vi "Build Array SB.vi"() -> ()   [LabVIEW 2019]
panel:
  out "Output Array":dbl[](array[numeric])
  in  "Index":i32
  in  "Element to Insert":dbl
  in  "Insert":bool
  in  "Stop":bool
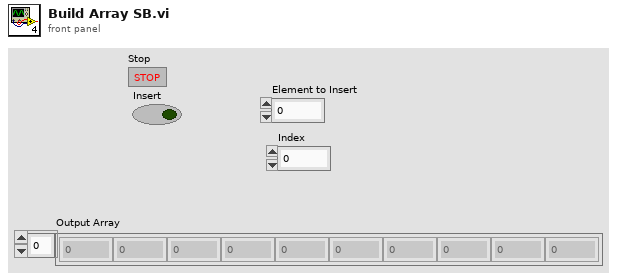
[diagram p1: front panel]
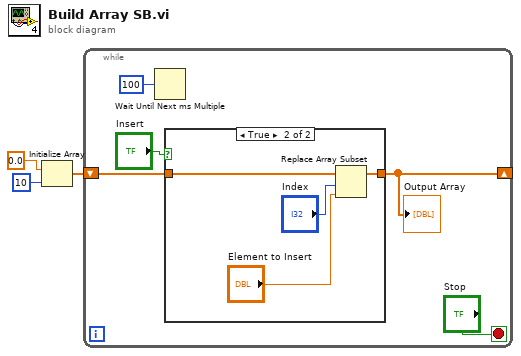
[diagram p0: block diagram]
diagram:
  n1 = Initialize Array(0.0 ("element"), 10 ("dimension size")) -> (w3:dbl[])
  n2 = while {
    shift-right: [w4] -> _
    shift-left: w3 -> [w5]
    stop <- "Stop" stop-if-true
    n3 = Wait Until Next ms Multiple(millisecond multiple=u32 100) -> ()  [unwired: 1 out]
    n4 = case shown="True" "Insert" {
      tunnel: [w9 w13] -> w4
      tunnel: w5 -> [w9 w12]
      frame False {
      }
      frame True {
        n5 = Replace Array Subset(array=w12, new element="Element to Insert", index="Index") -> (w13:dbl[])
      }
    }
    "Output Array" <- w4
  }
